vi "Dac_Output_cam_trig_synchronized_acquisition.vi"(0 "LabVIEW generated Sawtooth input":waveform(dbl)(graph)={"t0"=timestamp(0 s since 1904-01-01), "dt"=1.0, "Y"=array[1250 elements]}, 1 "Image acquisition time (ms)":dbl=100.0, 2 "Delay between frames (ms)":dbl=25.0) -> ()   [LabVIEW 2020]
uses:
  <vilib>/DAQmx/write.llb/DAQmx Write (Analog Wfm 1Chan NSamp).vi
  <vilib>/DAQmx/create/channels.llb/DAQmx Create Channel (AO-Voltage-Basic).vi
  <vilib>/DAQmx/configure/timing.llb/DAQmx Timing (Sample Clock).vi
  <vilib>/DAQmx/miscellaneous.llb/DAQmx Fill In Error Info.vi
  Global stop DAQ.vi
  <vilib>/DAQmx/create/channels.llb/DAQmx Create Channel (CO-Pulse Generation-Frequency).vi
  <vilib>/DAQmx/configure/timing.llb/DAQmx Timing (Implicit).vi
  <vilib>/DAQmx/configure/trigger.llb/DAQmx Start Trigger (Digital Edge).vi
  Global DAQ started.vi
  Global Counter count.vi
  <resource>/objmgr/daqmx.rc
  <vilib>/Utility/file.llb/Read Delimited Spreadsheet (DBL).vi
panel:
  in  "File to read":path=path "C:/Users/lpk27/Documents/ASLM/Image data/calibration_FPS_10_Flyback_25_ms.txt"
  out "CO.Count":u32=11249999
  in  "Setup":enum16{"Test setup", "Microscope"}(ring)=enum."Microscope"
  out "error out 4":errorcluster={"status"=TRUE, "code"=-200488, "source"="DAQmx Stop Task.vi:3590005<append>\n"}
  out "error out 3":errorcluster
  in  "error in":errorcluster
  out "# Samples written per channel":u32=1250
  out "actual frequency":dbl=10000.0
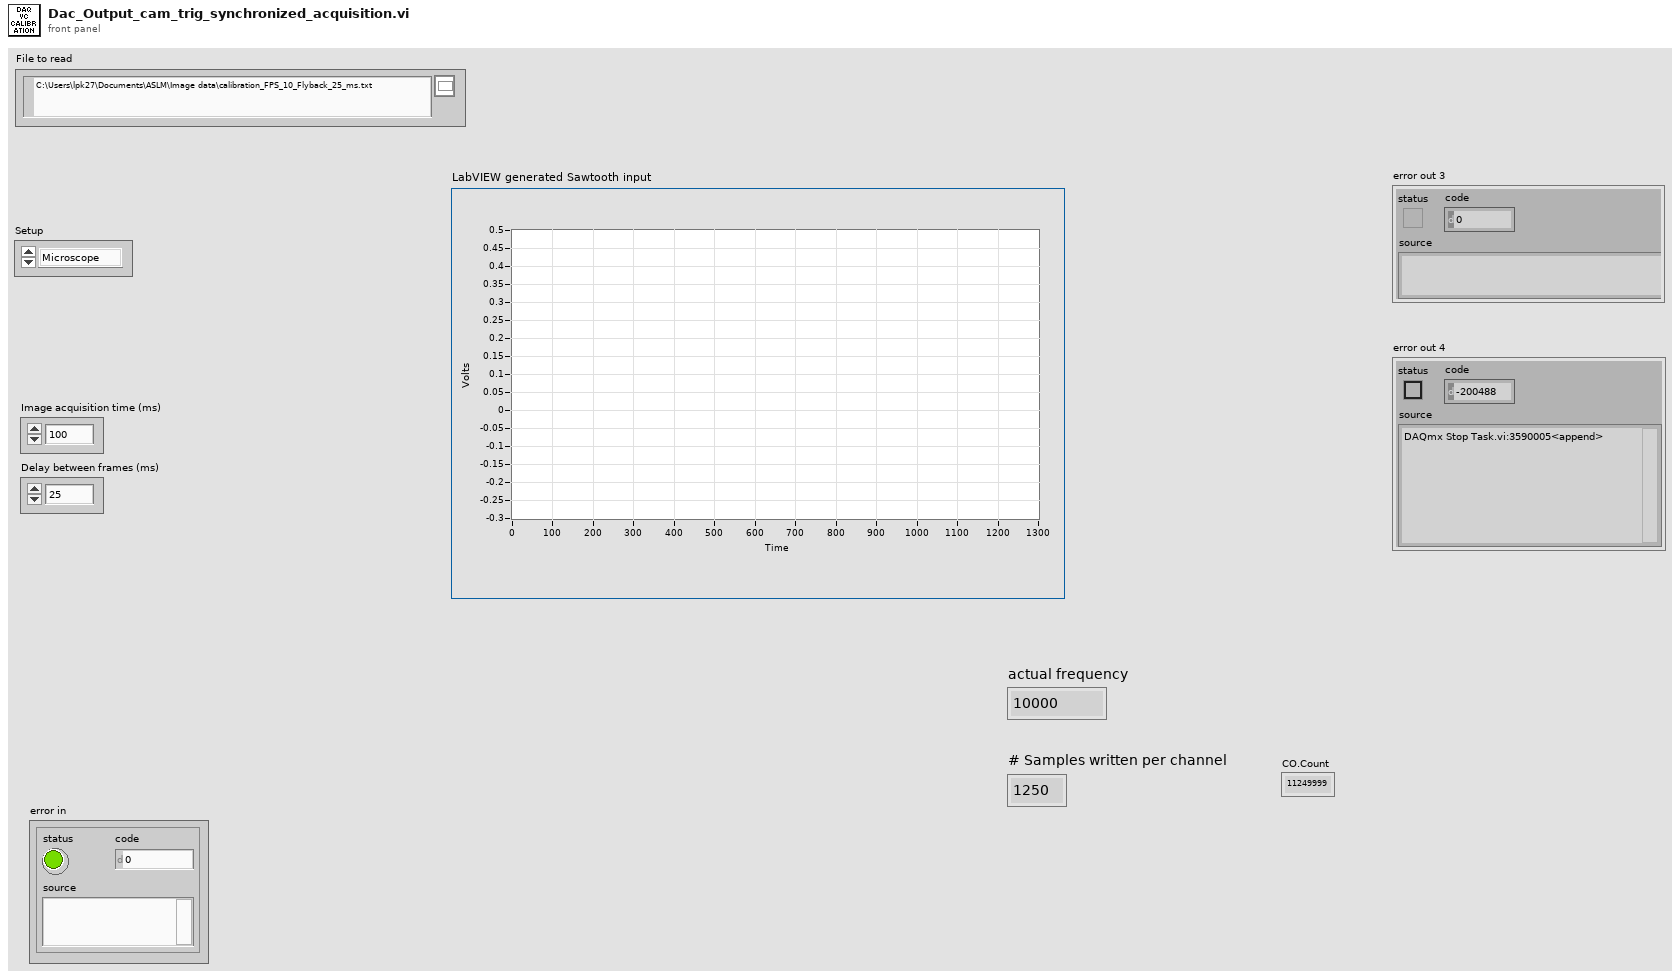
[diagram p1: front panel]
types:
  T1 = typedef "DAQ_channel_typedef.ctl" = cluster{"CO.Pulse.Term":tag, "Voice coil analog output":tag, "counter":tag, "CO.Pulse.Term 2":tag, "AOTF lines":tag, "counter 2":tag, "CO.Pulse.Term 3":tag, "counter 3":tag}
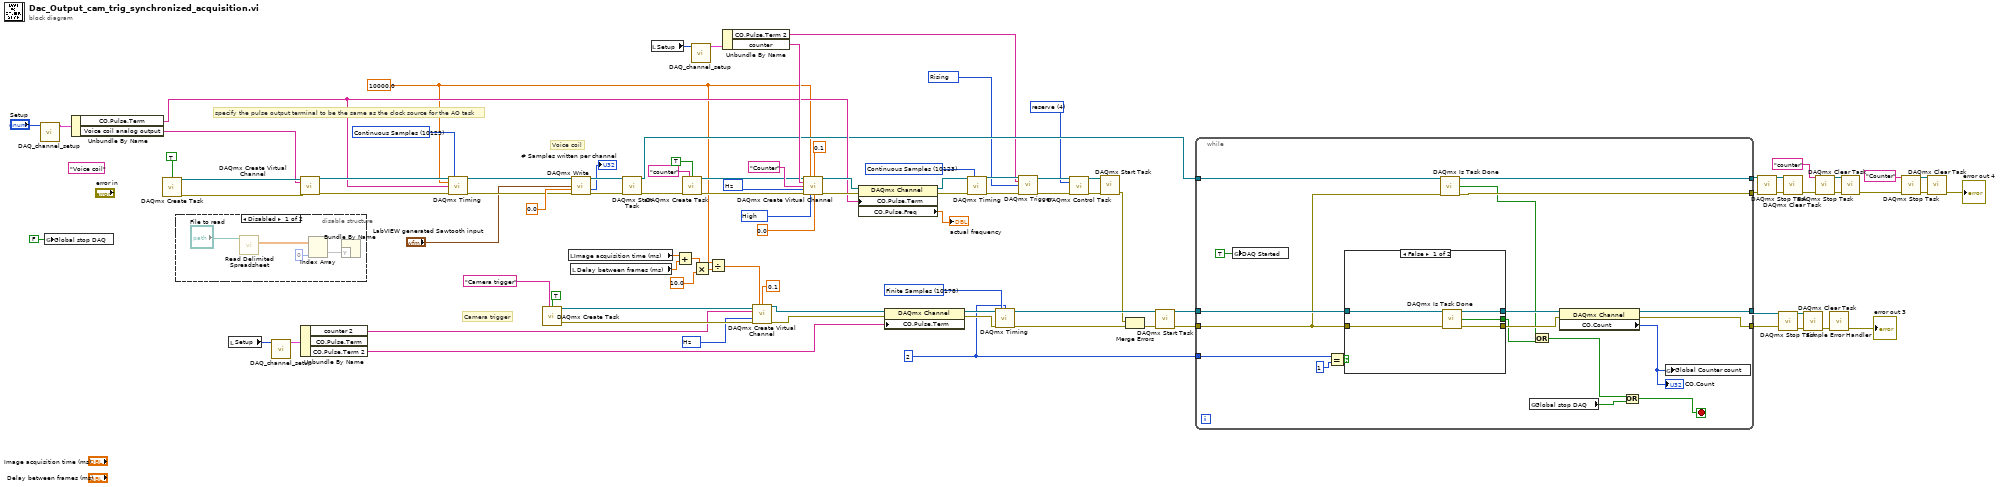
[diagram p0: block diagram]
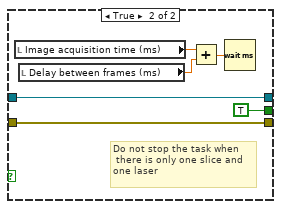
[diagram p3: hidden frame]
diagram:
  w2 = 2
  w9 = 4 items=["verify"=2, "reserve"=4, "commit"=3, "unreserve"=5, "abort"=6] ("action")
  w13 = 10280 items=["Rising"=10280, "Falling"=10171] ("edge")
  w22 = 10373 items=["Hz"=10373] ("units")
  (unwired) "Voice coil" ("new task name")
  w71 = 10178 items=["Finite Samples"=10178, "Continuous Samples"=10123, "Hardware Timed Single Point"=12522] ("sample mode")
  w82 = 10192 items=["High"=10192, "Low"=10214] ("idle state")
  w83 = 10373 items=["Hz"=10373] ("units")
  w76 = 10123 items=["Finite Samples"=10178, "Continuous Samples"=10123, "Hardware Timed Single Point"=12522] ("sample mode")
  w21 = 10000.0 ("rate")
  w93 = 10123 items=["Finite Samples"=10178, "Continuous Samples"=10123, "Hardware Timed Single Point"=12522] ("sample mode")
  # "Voice coil"
  # "Camera trigger"
  # "specify the pulse output terminal to be the same as the clock source for the AO task"
  n1 = call "DAQ_channel_setup.vi"("Text Ring"="Setup") -> ("DAQ channels OUT"=w42:T1)  [unwired: 10 in]
  n2 = global write "Global stop DAQ.vi" "Global stop DAQ"(FALSE ("Global stop DAQ")) -> ()
  n3 = Unbundle By Name(w42) -> ("CO.Pulse.Term"=w27:tag, "Voice coil analog output"=w43:tag)
  n4 = call <vilib>:"DAQmx Create Task.vi"("auto cleanup"=TRUE) -> ("task out"=w65:refnum<k21>, "error out"=w64:errorcluster)  [unwired: 13 in]
  n5 = disable-structure shown="Disabled" {
    frame Disabled {
      n6 = call-poly <vilib>:"Read Delimited Spreadsheet.vi"("file path (dialog if empty)"="File to read") -> ("all rows"=w98:dbl[][])  [unwired: 9 in, 5 out]
      n7 = Index Array(array=w98, index (col)=0 ("disabled index (col)")) -> (element=w96:dbl[])  [unwired: 1 in]
      n8 = Bundle By Name("Y"=w96) -> ()  [unwired: 1 in, 1 out]
    }
    frame Enabled {
    }
  }
  n9 = local read "Setup"() -> (w36:enum16{"Test setup", "Microscope"})
  n10 = call "DAQ_channel_setup.vi"("Text Ring"=w36) -> ("DAQ channels OUT"=w39:T1)  [unwired: 10 in]
  n11 = call-poly <vilib>:"DAQmx Create Virtual Channel.vi"("task in"=w65, "physical channels"=w43, "error in"=w64) -> ("task out"=w95:refnum<k21>, "error out"=w94:errorcluster)  [unwired: 11 in]
  n12 = Unbundle By Name(w39) -> ("counter 2"=w38:tag, "CO.Pulse.Term 2"=w3:tag)  [unwired: 1 out]
  n13 = call-poly <vilib>:"DAQmx Timing.vi"("task/channels in"=w95, "sample mode"=w93, "rate"=w21, "source"=w27, "error in"=w94) -> ("task out"=w78:refnum<k21>, "error out"=w77:errorcluster)  [unwired: 9 in]
  n14 = call <vilib>:"DAQmx Create Task.vi"("new task name"="Camera trigger", "auto cleanup"=TRUE) -> ("task out"=w62:refnum<k21>, "error out"=w63:errorcluster)  [unwired: 12 in]
  n15 = local read "Image acquisition time (ms)"() -> (w67:dbl)
  n16 = local read "Delay between frames (ms)"() -> (w66:dbl)
  n17 = call-poly <vilib>:"DAQmx Write.vi"("task/channels in"=w78, "data"="LabVIEW generated Sawtooth input", "timeout"=0.0, "error in"=w77) -> ("task out"=w87:refnum<k21>, "number of samples written per channel"=→"# Samples written per channel":u32, "error out"=w86:errorcluster)  [unwired: 9 in]
  n18 = call <vilib>:"DAQmx Start Task.vi"("task/channels in"=w87, "error in"=w86) -> ("task out"=w26:refnum<k21>, "error out"=w81:errorcluster)  [unwired: 12 in]
  n19 = local read "Setup"() -> (w35:enum16{"Test setup", "Microscope"})
  n20 = Add(x=w67, y=w66) -> (x+y=w18:dbl)
  n21 = call <vilib>:"DAQmx Create Task.vi"("new task name"="counter", "auto cleanup"=TRUE, "error in"=w81) -> ("task out"=w32:refnum<k21>, "error out"=w92:errorcluster)  [unwired: 11 in]
  n22 = call "DAQ_channel_setup.vi"("Text Ring"=w35) -> ("DAQ channels OUT"=w41:T1)  [unwired: 10 in]
  n23 = Multiply(x=w18, y=10.0) -> (x*y=w17:dbl)
  n24 = Divide(x=w21, y=w17) -> (x/y=w24:dbl)
  n25 = Unbundle By Name(w41) -> ("CO.Pulse.Term 2"=w12:tag, "counter"=w40:tag)
  n26 = call-poly <vilib>:"DAQmx Create Virtual Channel.vi"("task in"=w62, "frequency"=w24, "duty cycle"=0.1, "counter"=w38, "units"=w22, "error in"=w63) -> ("task out"=w75:refnum<k21>, "error out"=w69:errorcluster)  [unwired: 8 in]
  n27 = call-poly <vilib>:"DAQmx Create Virtual Channel.vi"("task in"=w32, "frequency"=w21, "duty cycle"=0.1, "counter"=w40, "name to assign"="Counter", "units"=w83, "error in"=w92, "idle state"=w82, "initial delay"=0.0) -> ("task out"=w91:refnum<k21>, "error out"=w90:errorcluster)  [unwired: 5 in]
  n28 = property class="DAQmx Channel"(reference=w91, error in=w90, "CO.Pulse.Term"=w27) -> (reference out=w88:refnum<k21>, error out=w89:errorcluster, "CO.Pulse.Freq"=→"actual frequency":dbl)
  n29 = property class="DAQmx Channel"(reference=w75, error in=w69, "CO.Pulse.Term"=w3) -> (reference out=w68:refnum<k21>, error out=w72:errorcluster)
  n30 = call-poly <vilib>:"DAQmx Timing.vi"("task/channels in"=w88, "sample mode"=w76, "error in"=w89) -> ("task out"=w15:refnum<k21>, "error out"=w14:errorcluster)  [unwired: 11 in]
  n31 = call-poly <vilib>:"DAQmx Timing.vi"("task/channels in"=w68, "sample mode"=w71, "samples per channel"=w2, "error in"=w72) -> ("task out"=w70:refnum<k21>, "error out"=w4:errorcluster)  [unwired: 10 in]
  n32 = call-poly <vilib>:"DAQmx Trigger.vi"("task/channels in"=w15, "source"=w12, "edge"=w13, "error in"=w14) -> ("task out"=w11:refnum<k21>, "error out"=w10:errorcluster)  [unwired: 10 in]
  n33 = call <vilib>:"DAQmx Control Task.vi"("task/channels in"=w11, "action"=w9, "error in"=w10) -> ("task out"=w8:refnum<k21>, "error out"=w7:errorcluster)  [unwired: 11 in]
  n34 = call <vilib>:"DAQmx Start Task.vi"("task/channels in"=w8, "error in"=w7) -> ("error out"=w5:errorcluster)  [unwired: 12 in, 1 out]
  n35 = Merge Errors(w5, w4) -> (w6:errorcluster)
  n36 = call <vilib>:"DAQmx Start Task.vi"("task/channels in"=w70, "error in"=w6) -> ("task out"=w74:refnum<k21>, "error out"=w73:errorcluster)  [unwired: 12 in]
  n37 = while {
    tunnel: w26 -> [w118]
    tunnel: w74 -> [w117]
    tunnel: w73 -> [w102]
    tunnel: [w116] -> w49
    tunnel: [w115] -> w48
    tunnel: [w111] -> w54
    tunnel: [w109] -> w53
    tunnel: w2 -> [w105]
    stop <- w106 stop-if-true
    n38 = global write "Global DAQ started.vi" "DAQ Started"(TRUE ("DAQ Started")) -> ()
    n39 = Equal?(x=w105, y=1) -> (x = y?=w103:bool)
    n40 = case shown="False" w103 {
      tunnel: w117 -> [w123 w129]
      tunnel: w102 -> [w122 w128]
      tunnel: [w121 w129] -> w112
      tunnel: [w120 w128] -> w110
      tunnel: [w119 TRUE ("task done?")] -> w107
      frame False {
        n41 = call <vilib>:"DAQmx Is Task Done.vi"("task/channels in"=w123, "error in"=w122) -> ("task out"=w121:refnum<k21>, "task done?"=w119:bool, "error out"=w120:errorcluster)  [unwired: 11 in]
      }
      frame True {
        # "Do not stop the task when\n there is only one slice and \none laser"
        n42 = local read "Image acquisition time (ms)"() -> (w125:dbl)
        n43 = local read "Delay between frames (ms)"() -> (w126:dbl)
        n44 = Add(x=w125, y=w126) -> (x+y=w124:dbl)
        n45 = Wait (ms)(milliseconds to wait=w124) -> ()  [unwired: 1 out]
      }
    }
    n46 = call <vilib>:"DAQmx Is Task Done.vi"("task/channels in"=w118, "error in"=w102) -> ("task out"=w116:refnum<k21>, "task done?"=w101:bool, "error out"=w115:errorcluster)  [unwired: 11 in]
    n47 = global read "Global stop DAQ.vi" "Global stop DAQ"() -> (w114:bool)
    n48 = Or(x=w101, y=w107) -> (x .or. y?=w100:bool)
    n49 = property class="DAQmx Channel"(reference=w112, error in=w110) -> (reference out=w111:refnum<k21>, error out=w109:errorcluster, "CO.Count"=w108:u32)
    "CO.Count" <- w108
    n50 = Or(x=w100, y=w114) -> (x .or. y?=w106:bool)
    n51 = global write "Global Counter count.vi" "Global Counter count"(w108) -> ()
  }
  n52 = call <vilib>:"DAQmx Stop Task.vi"("task/channels in"=w49, "error in"=w48) -> ("task out"=w52:refnum<k21>, "error out"=w51:errorcluster)  [unwired: 12 in]
  n53 = call <vilib>:"DAQmx Stop Task.vi"("task/channels in"=w54, "error in"=w53) -> ("task out"=w57:refnum<k21>, "error out"=w58:errorcluster)  [unwired: 12 in]
  n54 = call <vilib>:"DAQmx Clear Task.vi"("task in"=w52, "error in"=w51) -> ("error out"=w45:errorcluster)  [unwired: 13 in]
  n55 = call <vilib>:"DAQmx Clear Task.vi"("task in"=w57, "error in"=w58) -> ("error out"=w56:errorcluster)  [unwired: 13 in]
  n56 = call <vilib>:"DAQmx Stop Task.vi"("task/channels in"="counter" ("new task name"), "error in"=w45) -> ("task out"=w47:refnum<k21>, "error out"=w46:errorcluster)  [unwired: 12 in]
  n57 = call <vilib>:"Simple Error Handler.vi"("error in (no error)"=w56) -> ("error out"=→"error out 3":errorcluster)  [unwired: 4 in, 4 out]
  n58 = call <vilib>:"DAQmx Clear Task.vi"("task in"=w47, "error in"=w46) -> ("error out"=w44:errorcluster)  [unwired: 13 in]
  n59 = call <vilib>:"DAQmx Stop Task.vi"("task/channels in"="Counter" ("new task name"), "error in"=w44) -> ("task out"=w29:refnum<k21>, "error out"=w30:errorcluster)  [unwired: 12 in]
  n60 = call <vilib>:"DAQmx Clear Task.vi"("task in"=w29, "error in"=w30) -> ("error out"=→"error out 4":errorcluster)  [unwired: 13 in]
